vi "Init Match.vi"(4 "Not found":refnum<class "CConfig Query.lvclass">, 6 "Found":refnum<class "CConfig Query.lvclass">, 7 "Data [name]":string, 8 "error in (no error)":errorcluster) -> (0 "error out":errorcluster, 3 "Find First Query out":refnum<class "Loop Query.lvclass">)   [LabVIEW 2013, in "All Type Query.lvclass"]
doc: "Copyright 2018, Carya Automatisering, Wiebe Walstra."
uses:
  All Type Query.lvclass
  Loop Query.lvclass
  CConfig Query.lvclass
  All Type Query.lvclass/All Type Query.ctl
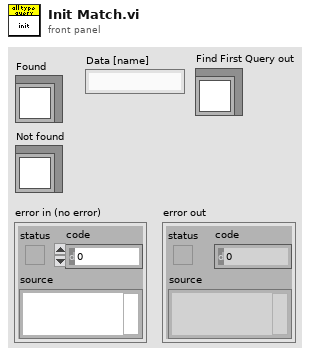
[diagram p1: front panel]
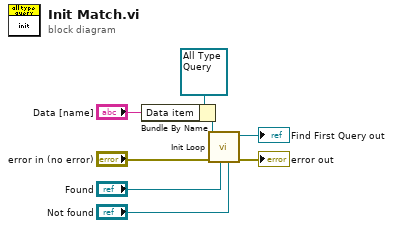
[diagram p0: block diagram]
diagram:
  n1 = Bundle By Name(cluster=refnum<class "All Type Query.lvclass"> refnum ("Find First Query in"), "Data item"="Data [name]") -> (w1:refnum<class "All Type Query.lvclass">)
  n2 = call "Init Loop.vi"("Not found"="Not found", "Found"="Found", "error in (no error)"="error in (no error)", "Loop Query"=w1) -> ("error out"=→"error out":errorcluster, "Loop Query"=→"Find First Query out":refnum<class "All Type Query.lvclass">)  [unwired: 6 in]
